vi "lib Degrees Arcmin Arcsec to Degrees decimal.vi"(8 "error in (no error)":errorcluster, 11 "Declination":T1) -> (0 "error out":errorcluster, 3 "Angle":dbl format="%#.8g")   [LabVIEW 2021]
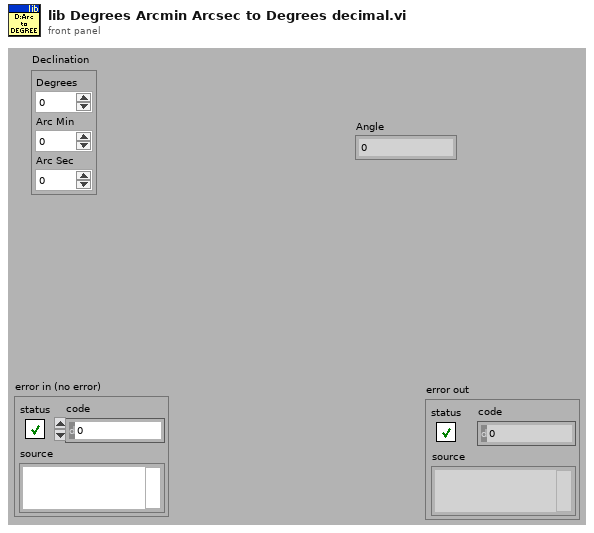
[diagram p1: front panel]
types:
  T1 = cluster{"Degrees":dbl, "Arc Min":dbl, "Arc Sec":dbl}
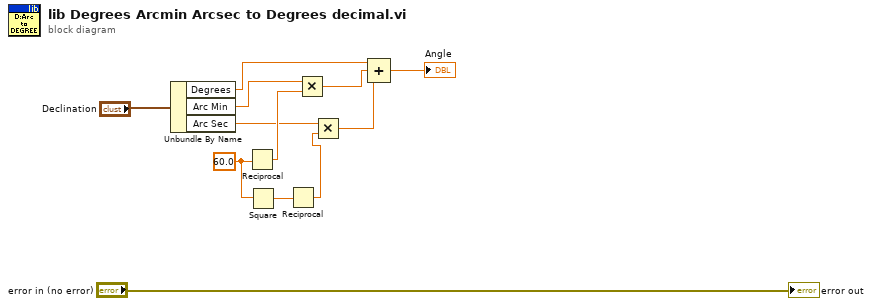
[diagram p0: block diagram]
diagram:
  w4 = 60.0
  n1 = Unbundle By Name("Declination") -> ("Degrees"=w9:dbl, "Arc Min"=w8:dbl, "Arc Sec"=w5:dbl)
  n2 = Reciprocal(x=w4) -> (1/x=w7:dbl)
  n3 = Square(x=w4) -> (x^2=w3:dbl)
  n4 = Reciprocal(x=w3) -> (1/x=w2:dbl)
  n5 = Multiply(x=w8, y=w7) -> (x*y=w6:dbl)
  n6 = Multiply(x=w5, y=w2) -> (x*y=w1:dbl)
  n7 = Compound Arithmetic op=ADD(w9, w6, w1) -> (→"Angle":dbl)
  "error out" <- "error in (no error)"
